vi "LCA Set Default Vel Unit.vi"(7 "Prefix":T3=-3 items=["UNIT"=0, "DECI"=-1, "CENTI"=-2, "MILLI"=-3, "MICRO"=-6], 8 "error in (no error)":errorcluster caption="Fehler (Eingang, kein Fehler)", 9 "TimeUnit":T1=1 items=["PER_SECOND"=1, "PER_MINUTE"=60, "PER_HOUR"=3600], 10 "Position Unit":T2 items=["METERS", "REVOLUTIONS", "DEGREE", "RADIAN", "DEVICE"], 11 "Axis Handle":i64) -> (0 "error out":errorcluster caption="Fehler (Ausgang)")   [LabVIEW 2021, in "labbCAN_MotionControl_API.lvlib"]
doc: "LCA_Func long __stdcall LCA_SetDefaultVelUnit(dev_hdl hAxis,\n char Prefix,\n int PositionUnit,\n int TimeUnit);"
uses:
  labbCAN_MotionControl_API.lvlib
  labbCAN_Bus_API/SiUnitPrefix.ctl
  PositionUnits.ctl
  labbCAN_Bus_API/TimeUnits.ctl
  labbCAN_MotionControl_API.dll
  labbCAN_Bus_API/labbCAN_Bus_API.lvlib
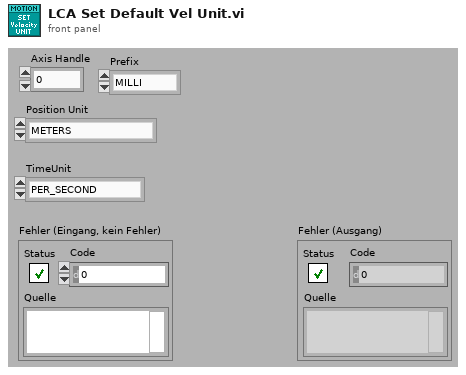
[diagram p1: front panel]
types:
  T1 = typedef "labbCAN_Bus_API.lvlib/TimeUnits.ctl" = i32
  T2 = typedef "labbCAN_MotionControl_API.lvlib/PositionUnits.ctl" = i32
  T3 = typedef "labbCAN_Bus_API.lvlib/SiUnitPrefix.ctl" = i32
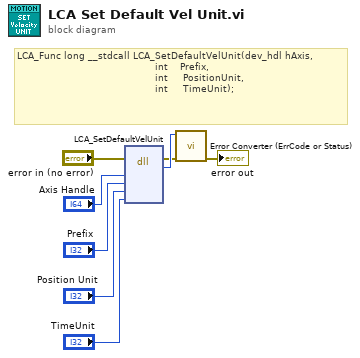
[diagram p0: block diagram]
diagram:
  # "LCA_Func long __stdcall LCA_SetDefaultVelUnit(dev_hdl hAxis,\n                                              int    Prefix,\n                                              int     PositionUnit,\n                                              int     TimeUnit);"
  n1 = dll-call lib="C:/Users/olaja/AppData/Local/CETONI_SDK/labbCAN_MotionControl_API.*" fn="LCA_SetDefaultVelUnit"(error in="error in (no error)", "hAxis"="Axis Handle", "Prefix"="Prefix", "PositionUnit"="Position Unit", "TimeUnit"="TimeUnit") -> (error out=w2:errorcluster, "Rückgabetyp"=w8:i32)  [unwired: 6 in, 1 out]
  n2 = call "Error Converter (ErrCode or Status).vi"("error in (no error)"=w2, "error code"=w8) -> ("error out"=→"error out":errorcluster)  [unwired: 9 in]
